vi "Deadband.vi"(10 "Inputs":dbl[](array[numeric]), 11 "Deadband":dbl) -> (3 "Ouptuts":dbl[](array[numeric]))   [LabVIEW 2020]
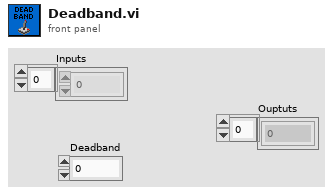
[diagram p1: front panel]
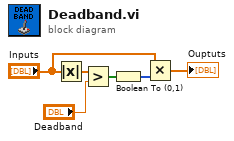
[diagram p0: block diagram]
diagram:
  n1 = Absolute Value(x="Inputs") -> (abs(x)=w2:dbl[])
  n2 = Greater?(x=w2, y="Deadband") -> (0:w4:bool[])
  n3 = Boolean To (0,1)(Boolean=w4) -> (0, 1=w5:i16[])
  n4 = Multiply(x="Inputs", y=w5) -> (x*y=→"Ouptuts":dbl[])
